vi "Write Limits.vi"(8 "error in (no error)":errorcluster, 10 "Limits":T1, 11 "Alarms in":refnum<class "HK Alarms.lvclass">) -> (0 "error out":errorcluster, 3 "Alarms out":refnum<class "HK Alarms.lvclass">)   [LabVIEW 2019, in "HK Alarms.lvclass"]
uses:
  HK Alarms/HK Alarms.lvclass
  HK Item/HK Channel Settings Limits.ctl
  HK Alarms/HK Alarms.lvclass/HK Alarms.ctl
  HK Item/HK Item.lvclass
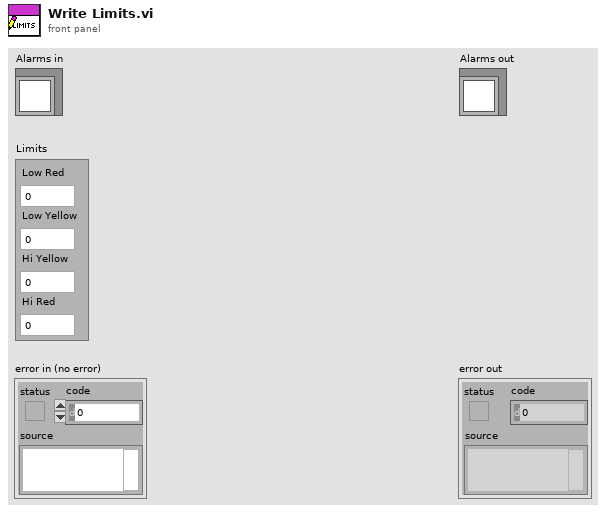
[diagram p1: front panel]
types:
  T1 = typedef "HK Item.lvclass/HK Channel Settings Limits.ctl" = cluster{"Low Red":dbl, "Low Yellow":dbl, "Hi Yellow":dbl, "Hi Red":dbl}
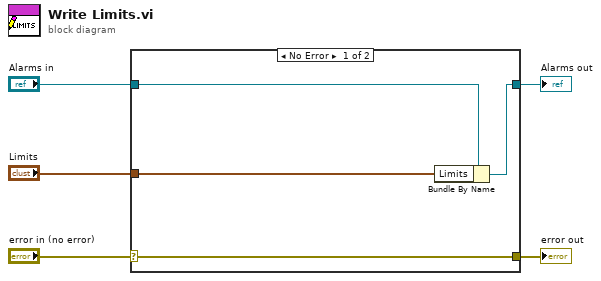
[diagram p0: block diagram]
diagram:
  n1 = case shown="No Error" "error in (no error)" {
    selector: "error in (no error)" -> [w9 w10]
    tunnel: [w9 w10] -> w4
    tunnel: [w7 w11] -> w2
    tunnel: "Alarms in" -> [w8 w11]
    tunnel: "Limits" -> [w6 _]
    frame No Error {
      n2 = Bundle By Name(cluster=w8, "Limits"=w6) -> (w7:refnum<class "HK Alarms.lvclass">)
    }
    frame Error {
    }
  }
  "error out" <- w4
  "Alarms out" <- w2
